vi "Untitled 1.vi"() -> (0 "error out":errorcluster, 2 "Array":T1(array[cluster]))   [LabVIEW 2014, in "SetUp VIs.lvlib"]
uses:
  SetUp VIs.lvlib
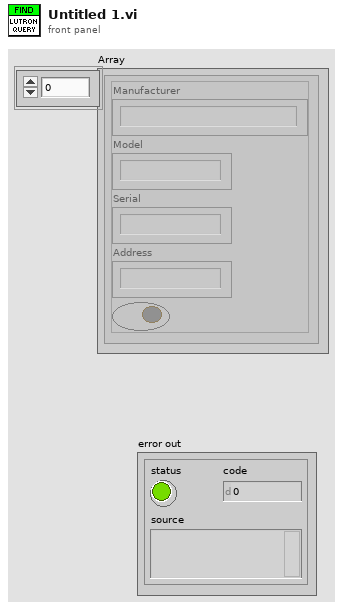
[diagram p1: front panel]
types:
  T1 = cluster{"Manufacturer":string, "Model":string, "Serial":string, "Address":string, "Boolean":bool}[]
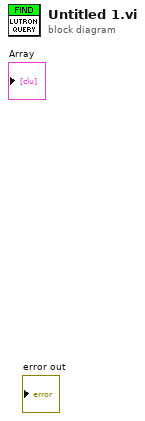
[diagram p0: block diagram]
diagram:
